vi "Close NI-Digital Session.vi"(8 "error in (no error)":errorcluster, 10 "session information":T1, 11 "instrument handle":refnum<k15>) -> (0 "error out":errorcluster)   [LabVIEW 2020, in "NIDigitalSPI.lvlib"]
doc: "Closes the given NI-DCPower instrument handle."
uses:
  NIDigitalSPI.lvlib
  <vilib>/MeasurementLink/MeasurementLink Session Management Client/RPC Messages/ni_measurementlink_sessionmanagement_v1_SessionInformation.ctl
  <vilib>/MeasurementLink/MeasurementLink Session Management Client/RPC Messages/nidevice_grpc_Session.ctl
  <vilib>/MeasurementLink/MeasurementLink Session Management Client/RPC Messages/ni_measurementlink_sessionmanagement_v1_ChannelMapping.ctl
  <vilib>/MeasurementLink/MeasurementLink Session Management Client/MeasurementLink Session Management Client.lvlib
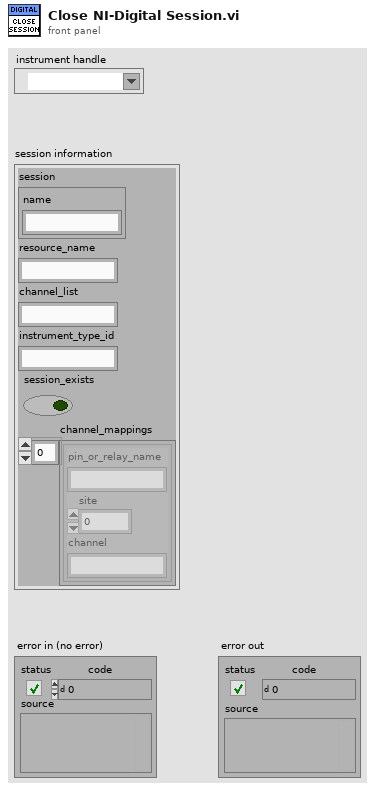
[diagram p1: front panel]
types:
  T1 = typedef "MeasurementLink Session Management Client.lvlib/ni_measurementlink_sessionmanagement_v1_SessionInformation.ctl" = cluster{"session":T2, "resource_name":string, "channel_list":string, "instrument_type_id":string, "session_exists":bool, "channel_mappings":T3[]}
  T2 = typedef "MeasurementLink Session Management Client.lvlib/nidevice_grpc_Session.ctl" = cluster{"name":string}
  T3 = typedef "MeasurementLink Session Management Client.lvlib/ni_measurementlink_sessionmanagement_v1_ChannelMapping.ctl" = cluster{"pin_or_relay_name":string, "site":i32, "channel":string}
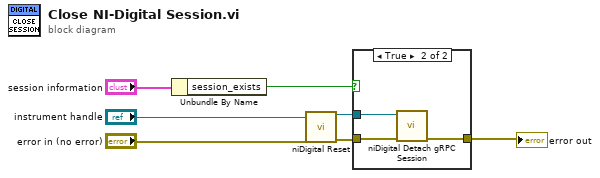
[diagram p0: block diagram]
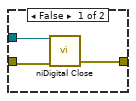
[diagram p2: hidden frame]
diagram:
  n1 = Unbundle By Name("session information") -> ("session_exists"=w2:bool)
  n2 = call <instrlib>:"niDigital Reset.vi"("instrument handle in"="instrument handle", "error in"="error in (no error)") -> ("instrument handle out"=w3:refnum<k15>, "error out"=w4:errorcluster)  [unwired: 12 in]
  n3 = case shown="True" w2 {
    tunnel: w3 -> [w10 w11]
    tunnel: w4 -> [w9 w12]
    tunnel: [w8 w13] -> w6
    frame False {
      n4 = call <instrlib>:"niDigital Close.vi"("instrument handle"=w10, "error in"=w9) -> ("error out"=w8:errorcluster)  [unwired: 13 in]
    }
    frame True {
      n5 = call <instrlib>:"niDigital Detach gRPC Session.vi"("instrument handle"=w11, "error in"=w12) -> ("error out"=w13:errorcluster)  [unwired: 13 in]
    }
  }
  "error out" <- w6
